vi "Close.vi"(8 "Error In":errorcluster) -> (0 "Error Out":errorcluster)   [LabVIEW 2011, in "LVH-Interface-for-Kinect.lvlib"]
uses:
  <vilib>/LabVIEW Hacker/LVH-Interface-for-Kinect/LVH-Interface-for-Kinect.lvlib
  <vilib>/LabVIEW Hacker/LVH-Interface-for-Kinect/Public/lib/freenect_sync.dll
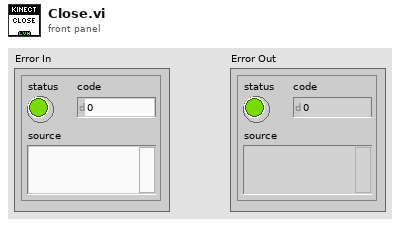
[diagram p1: front panel]
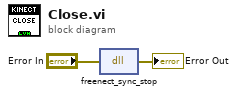
[diagram p0: block diagram]
diagram:
  n1 = dll-call lib="C:/Program Files (x86)/National Instruments/LabVIEW 2011/vi.lib/LabVIEW Hacker/LVH-Interface-for-Kinect/Public/lib/freenect_sync.dll" fn="freenect_sync_stop"(error in="Error In") -> (error out=→"Error Out":errorcluster)  [unwired: 3 in, 1 out]
